vi "QHM Demo_Template.vi"(11 "Sender":string="demo") -> ()   [LabVIEW 2014]
uses:
  <vilib>/Utility/miscctls.llb/LVPointTypeDef.ctl
panel:
  out "optput":T1
  in  "Creat error":bool
  in  "log":i32(listbox)
  in  "Quit":bool
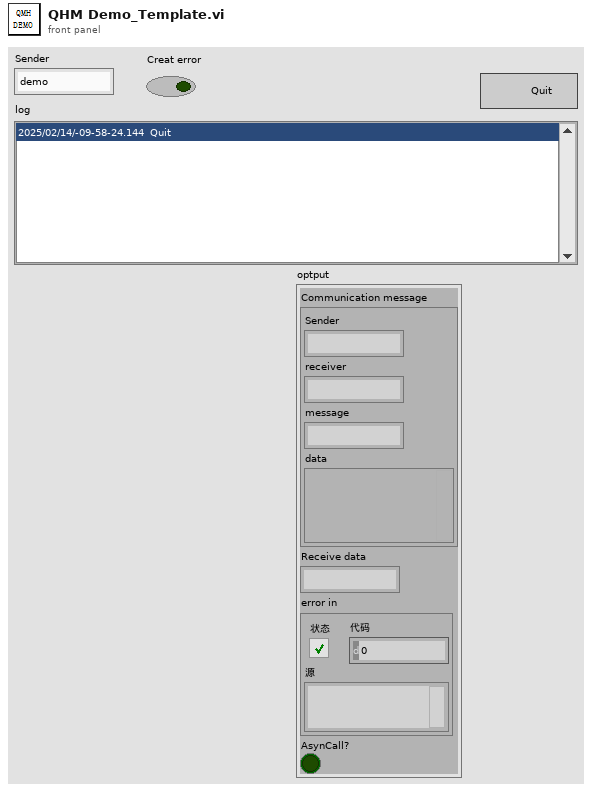
[diagram p1: front panel]
types:
  T1 = cluster{"Communication message":cluster{"Sender":string, "receiver":string, "message":string, "data":variant}, "Receive data":string, "error in":errorcluster, "AsynCall?":bool}
  T2 = cluster{"Sender":string, "receiver":string, "message":string, "data":variant}
  T3 = typedef "LVPointTypeDef.ctl" = cluster{"Horizontal":i16, "Vertical":i16}
  T4 = enum32{"invalid app kind", "Development System", "Run Time System", "Student Edition", "Embedded LabVIEW", "Evaluation", "Custom"}
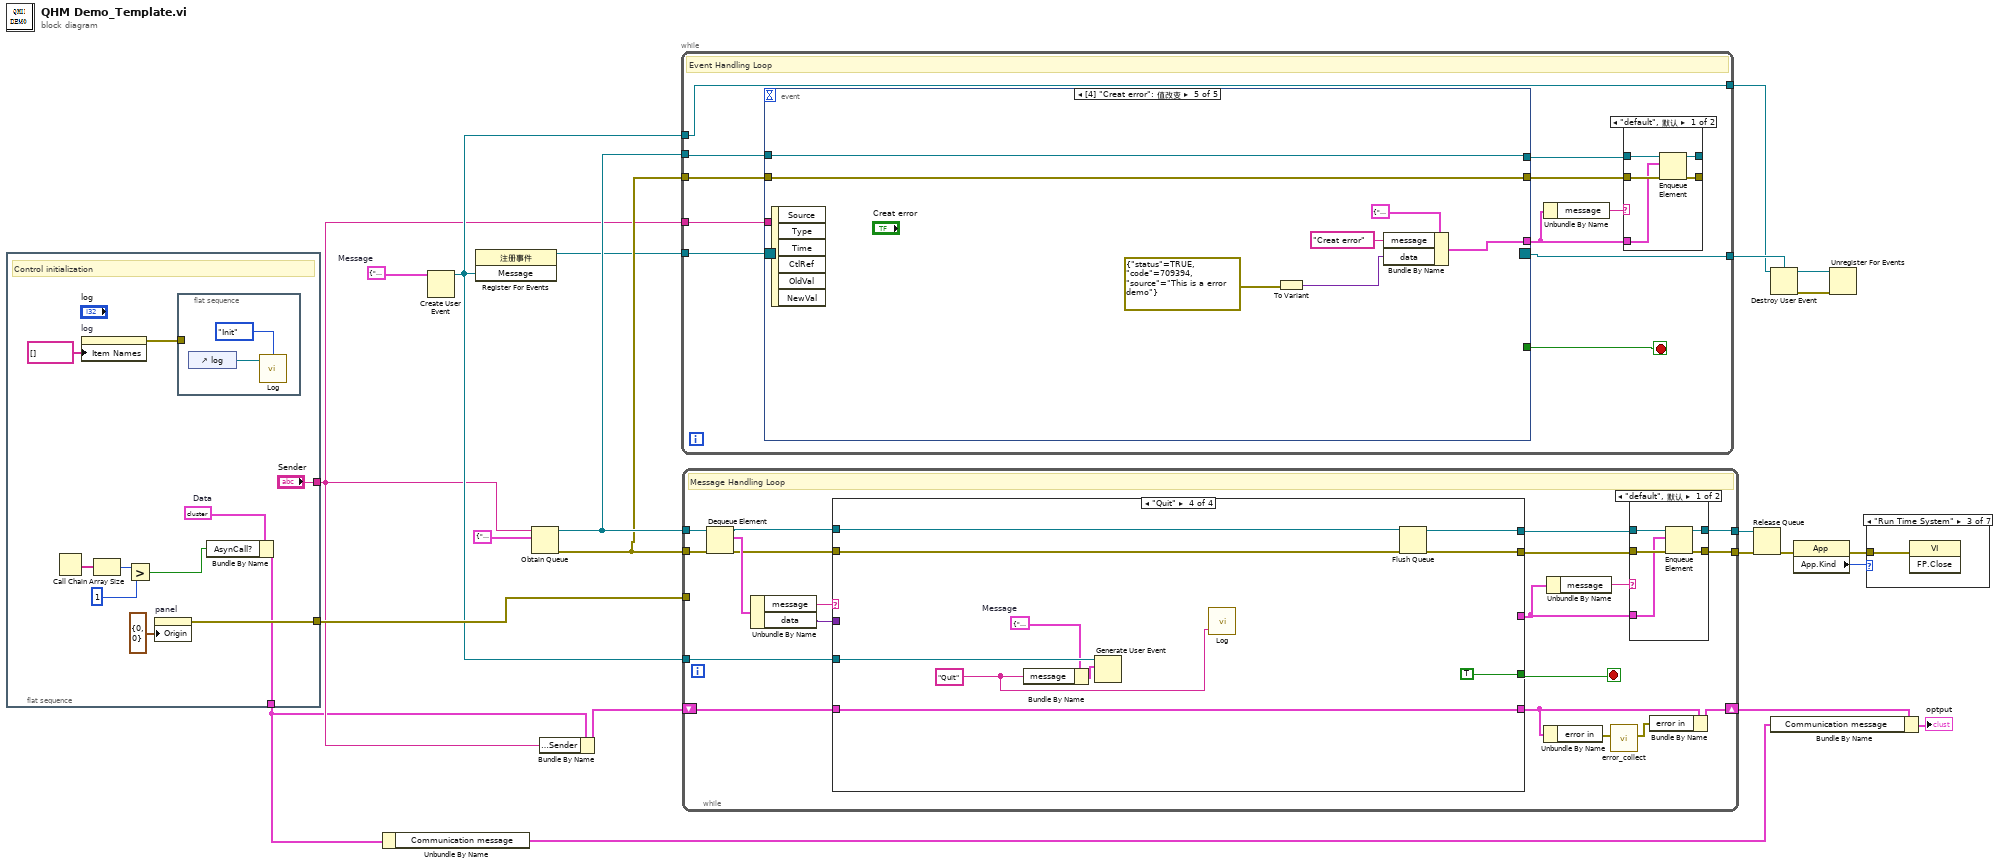
[diagram p0: block diagram]
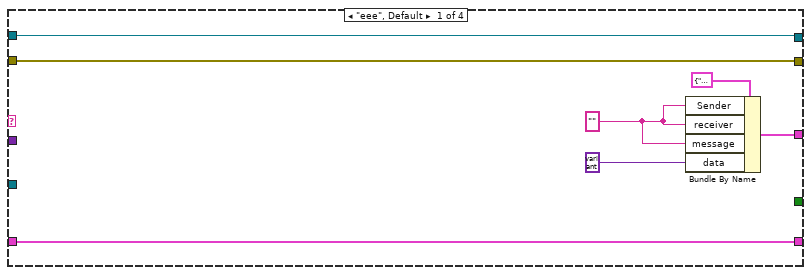
[diagram p9: hidden frame]
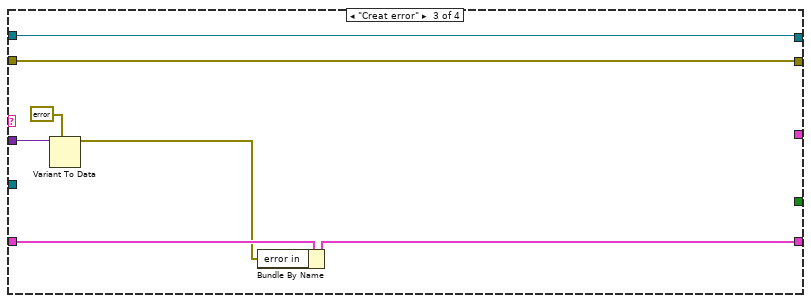
[diagram p11: hidden frame]
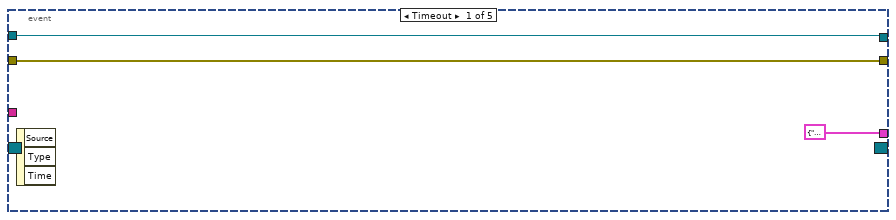
[diagram p13: hidden frame]
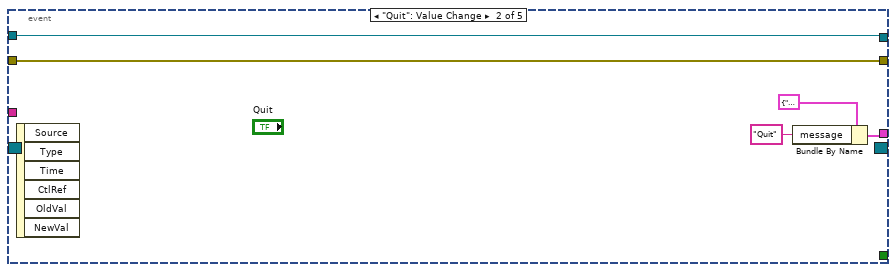
[diagram p14: hidden frame]
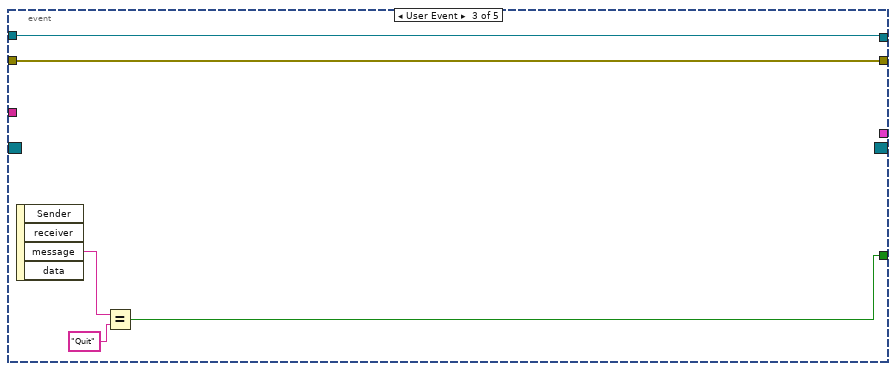
[diagram p15: hidden frame]
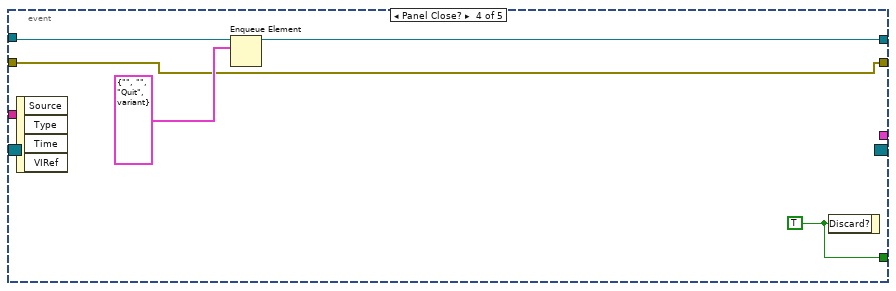
[diagram p16: hidden frame]
diagram:
  w1 = T2 {"Sender"="", "receiver"="", "message"="", "data"=variant}  # Message
  n1 = flat-sequence {
    tunnel: [w31] -> w11
    tunnel: ["Sender"] -> w4
    tunnel: [w24] -> w3
    frame #0 {
      w25 = T1 {"Communication message"={"Sender"="", "receiver"="", "message"="", "data"=variant}, "Receive data"="", "error in"={"status"=FALSE, "code"=0, "source"=""}, "AsynCall?"=FALSE}  # Data
      # "Control initialization"
      n2 = Call Chain() -> (call chain=w26:string[])
      n3 = property on="log" class="LstBox (严格)"("Item Names"=string[] [] ("项名")) -> (error out=w29:errorcluster)  [unwired: 2 in, 1 out]
      n4 = Array Size(array=w26) -> (size(s)=w28:i32)
      n5 = Greater?(x=w28, y=1) -> (0:w23:bool)
      n6 = property on="panel" class="Pane"("Origin"=T3 {"Horizontal"=0, "Vertical"=0} ("原点")) -> (error out=w31:errorcluster)  [unwired: 2 in, 1 out]
      n7 = flat-sequence {
        tunnel: w29 -> [_]
        frame #0 {
          n8 = control-ref of="log"() -> (w33:refnum<vi>)
          n9 = call "Log.vi"("Method"=enum16{"Init", "Log"}."Init", "ListBox in"=w33) -> ()  [unwired: 2 in]
        }
      }
      n10 = Bundle By Name(cluster=w25, "AsynCall?"=w23) -> (w24:T1)
    }
  }
  n11 = Unbundle By Name(w3) -> ("Communication message"=w5:T2)
  n12 = Create User Event(user event datatype=w1) -> (user event=w8:refnum<user-event>)  [unwired: 1 in, 1 out]
  n13 = register-events(w8) -> (reference out=w12:refnum<event-registration>)  [unwired: 2 in, 1 out]
  n14 = Obtain Queue(name (unnamed)=w4, element data type=T2 {"Sender"="", "receiver"="", "message"="", "data"=variant} ("Communication message")) -> (queue out=w21:refnum<queue>, error out=w14:errorcluster)  [unwired: 3 in, 1 out]
  n15 = Bundle By Name(cluster=w3, "Communication message.Sender"=w4) -> (w13:T1)
  n16 = while {
    tunnel: w21 -> [w44]
    tunnel: w14 -> [w42]
    tunnel: w4 -> [w38]
    tunnel: w12 -> [w37]
    tunnel: [w36] -> w10
    tunnel: w8 -> [w35]
    tunnel: [w35] -> w7
    stop <- w45 stop-if-true
    # "Event Handling Loop"
    n17 = event shown="[4] \"Creat error\": 值改变" {
      selector: w37 -> [_ _ _ _ _]
      dyn-events: [_ _ _ _ _] -> w36
      timeout: _ -> [_ _ _ _ _]
      tunnel: [_ _ w63 w67 _] -> w45
      tunnel: w44 -> [w55 w60 w65 w70 w77]
      tunnel: [w55 w60 w65 w68 w77] -> w43
      tunnel: [T2 {"Sender"="", "receiver"="", "message"="", "data"=variant} ("Communication message") w59 _ _ w73] -> w40
      tunnel: [w54 w58 w62 w66 w76] -> w41
      tunnel: w42 -> [w54 w58 w62 w66 w76]
      tunnel: w38 -> [_ _ _ _ _]
      event Timeout {
        n18 = event-data() -> ()  [unwired: 1 in, 3 out]
      }
      event "Quit": Value Change {
        n19 = event-data() -> ()  [unwired: 1 in, 6 out]
        n20 = Bundle By Name(cluster=T2 {"Sender"="", "receiver"="", "message"="", "data"=variant} ("Communication message"), "message"="Quit" ("Sender")) -> (w59:T2)
      }
      event User Event {
        n21 = event-data() -> ("message"=w61:string)  [unwired: 1 in, 3 out]
        n22 = Equal?(x=w61, y="Quit") -> (x = y?=w63:bool)
      }
      event Panel Close? {
        w67 = TRUE ("放弃？")
        n23 = event-data() -> ()  [unwired: 1 in, 4 out]
        n24 = Enqueue Element(queue=w70, element=T2 {"Sender"="", "receiver"="", "message"="Quit", "data"=variant} ("Communication message")) -> (queue out=w68:refnum<queue>)  [unwired: 2 in, 2 out]
        n25 = event-data("Discard?"=w67) -> ()  [unwired: 1 in, 1 out]
      }
      event "Creat error": Value Change {
        n26 = event-data() -> ()  [unwired: 1 in, 6 out]
        n27 = To Variant(anything=errorcluster {"status"=TRUE, "code"=709394, "source"="This is a error demo"}) -> (Variant=w71:variant)
        n28 = Bundle By Name(cluster=T2 {"Sender"="", "receiver"="", "message"="", "data"=variant} ("Communication message"), "message"="Creat error" ("Sender"), "data"=w71) -> (w73:T2)
      }
    }
    n29 = Unbundle By Name(w40) -> ("message"=w39:string)
    n30 = case shown="\"default\", 默认" w39 {
      tunnel: w43 -> [w50 w52]
      tunnel: w41 -> [w49 w51]
      tunnel: w40 -> [w48 _]
      tunnel: [w47 w52] -> _
      tunnel: [w46 w51] -> _
      frame "default", Default {
        n31 = Enqueue Element(queue=w50, element=w48, error in (no error)=w49) -> (queue out=w47:refnum<queue>, error out=w46:errorcluster)  [unwired: 1 in, 1 out]
      }
      frame "" {
      }
    }
  }
  n32 = while {
    tunnel: w21 -> [w97]
    tunnel: w14 -> [w96]
    tunnel: [w88] -> w20
    tunnel: [w87] -> w19
    shift-right: [w79] -> w6
    shift-left: w13 -> [w83]
    tunnel: w11 -> [_]
    tunnel: w8 -> [w82]
    stop <- w86 stop-if-true
    # "Message Handling Loop"
    n33 = Dequeue Element(queue=w97, error in (no error)=w96) -> (queue out=w93:refnum<queue>, element=w95:T2, error out=w92:errorcluster)  [unwired: 1 in, 1 out]
    n34 = Unbundle By Name(w95) -> ("message"=w94:string, "data"=w89:variant)
    n35 = case shown="\"Quit\"" w94 {
      tunnel: [w111 w114 w121 w130] -> w91
      tunnel: w93 -> [w111 w114 w121 w129]
      tunnel: w92 -> [w110 w113 w120 w127]
      tunnel: [w110 w113 w120 w128] -> w90
      tunnel: w89 -> [_ _ w118 _]
      tunnel: [_ _ _ TRUE] -> w86
      tunnel: [w108 _ _ _] -> w85
      tunnel: [w105 w112 w116 w126] -> w81
      tunnel: w83 -> [w105 w112 w119 w126]
      tunnel: w82 -> [_ _ _ w125]
      frame "eee", Default {
        w106 = ""
        n36 = Bundle By Name(cluster=T2 {"Sender"="", "receiver"="", "message"="", "data"=variant} ("Communication message"), "Sender"=w106, "receiver"=w106, "message"=w106, "data"=variant) -> (w108:T2)
      }
      frame "Init" {
      }
      frame "Creat error" {
        n37 = Variant To Data(type=errorcluster {"status"=FALSE, "code"=0, "source"=""} ("error out"), Variant=w118) -> (data=w115:errorcluster)  [unwired: 1 in, 1 out]
        n38 = Bundle By Name(cluster=w119, "error in"=w115) -> (w116:T1)
      }
      frame "Quit" {
        w124 = T2 {"Sender"="", "receiver"="", "message"="", "data"=variant}  # Message
        w122 = "Quit" ("y")
        n39 = Bundle By Name(cluster=w124, "message"=w122) -> (w123:T2)
        n40 = Generate User Event(user event=w125, event data cluster=w123) -> ()  [unwired: 2 in, 2 out]
        n41 = call "Log.vi"("Data"=w122) -> ()  [unwired: 3 in]
        n42 = Flush Queue(queue=w129, error in (no error)=w127) -> (queue out=w130:refnum<queue>, error out=w128:errorcluster)  [unwired: 1 out]
      }
    }
    n43 = Unbundle By Name(w81) -> ("error in"=w80:errorcluster)
    n44 = Unbundle By Name(w85) -> ("message"=w84:string)
    n45 = call "error_collect.vi"("error in (no error)"=w80) -> ("error IO"=w78:errorcluster)  [unwired: 10 in]
    n46 = case shown="\"default\", 默认" w84 {
      tunnel: w91 -> [w102 w104]
      tunnel: w90 -> [w101 w103]
      tunnel: w85 -> [w100 _]
      tunnel: [w99 w104] -> w88
      tunnel: [w98 w103] -> w87
      frame "default", Default {
        n47 = Enqueue Element(queue=w102, element=w100, error in (no error)=w101) -> (queue out=w99:refnum<queue>, error out=w98:errorcluster)  [unwired: 1 in, 1 out]
      }
      frame "" {
      }
    }
    n48 = Bundle By Name(cluster=w81, "error in"=w78) -> (w79:T1)
  }
  n49 = Release Queue(queue=w20, error in (no error)=w19) -> (error out=w18:errorcluster)  [unwired: 1 in, 2 out]
  n50 = Destroy User Event(user event=w7) -> (error out=w9:errorcluster)  [unwired: 1 in]
  n51 = Bundle By Name(cluster=w6, "Communication message"=w5) -> (→"optput":T1)
  n52 = property class="App"(error in=w18) -> (error out=w17:errorcluster, "App.Kind"=w16:T4)  [unwired: 1 in, 1 out]
  n53 = Unregister For Events(event registration refnum=w10, error in=w9) -> ()  [unwired: 1 out]
  n54 = case shown="\"Run Time System\"" w16 {
    tunnel: w17 -> [_ _ w132 _ _ _ _]
    frame "invalid app kind", Default {
    }
    frame "Development System" {
    }
    frame "Run Time System" {
      n55 = invoke class="VI" method="FP.Close"(error in=w132) -> ()  [unwired: 2 in, 3 out]
    }
    frame "Student Edition" {
    }
    frame "Embedded LabVIEW" {
    }
    frame "Evaluation" {
    }
    frame "Custom" {
    }
  }
